vi "M01 Wind Turbine.vi"(11 "EV3 in":T1) -> ()   [LabVIEW 2016]
uses:
  <vilib>/NXT/Subs/LVHSConnector.ctl
  <vilib>/NXT/LegoClasses/BrickReference/BrickReference.lvclass
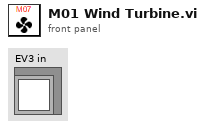
[diagram p1: front panel]
types:
  T1 = typedef "LVHSConnector.ctl" = refnum<class "BrickReference.lvclass">
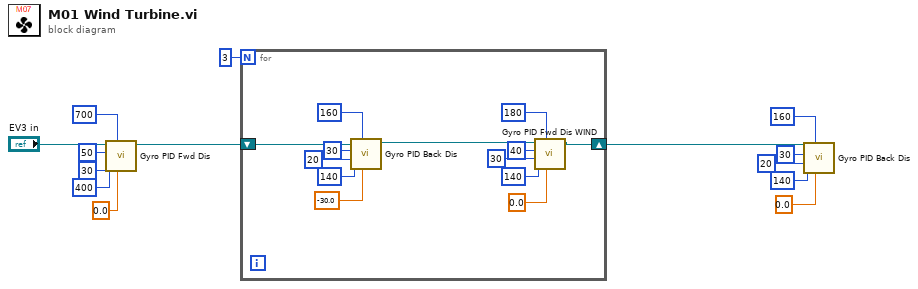
[diagram p0: block diagram]
diagram:
  n1 = call "Gyro PID Fwd Dis.vi"("Target angle"=sgl 0.0, "Threshold to stop"=700, "Threshold to slow"=400, "Min. speed"=30, "Max. speed"=50, "EV3 in"="EV3 in") -> ("EV3 out"=w7:T1)  [unwired: 5 in]
  n2 = for {
    N: 3 -> [_]
    shift-right: [w17] -> w8
    shift-left: w7 -> [w16]
    n3 = call "Gyro PID Back Dis.vi"("Target angle"=sgl -30.0, "Threshold to stop"=160, "Threshold to slow"=140, "Min. speed"=20, "Max. speed"=30, "EV3 in"=w16) -> ("EV3 out"=w18:T1)  [unwired: 5 in]
    n4 = call "Gyro PID Fwd Dis WIND.vi"("Target angle"=sgl 0.0, "Threshold to stop"=180, "Threshold to slow"=140, "Higher speed"=30, "Max. speed"=40, "EV3 in"=w18) -> ("EV3 out"=w17:T1)  [unwired: 5 in]
  }
  n5 = call "Gyro PID Back Dis.vi"("Target angle"=sgl 0.0, "Threshold to stop"=160, "Threshold to slow"=140, "Min. speed"=20, "Max. speed"=30, "EV3 in"=w8) -> ()  [unwired: 5 in, 1 out]
